vi "0008_FireEveryLastDayOfMonth.vi"(8 "error in (no error)":errorcluster) -> (0 "error out":errorcluster)   [LabVIEW 2013]
uses:
  <vilib>/addons/_JKI Toolkits/Caraya/classes/Assert/Assert True.vi
  source/Cron/Create Cron Expression.vi
  source/Cron/Compute Next Cron.vi
  source/Cron.Quartz/Cron.Quartz.lvclass
  <vilib>/addons/_JKI Toolkits/Caraya/classes/Test/Test.lvclass
  <vilib>/addons/_JKI Toolkits/Caraya/classes/Assert/Assert.lvclass
  source/openCron.lvlib
panel:
  out "Occurences":timestamp[](array[timestamp])
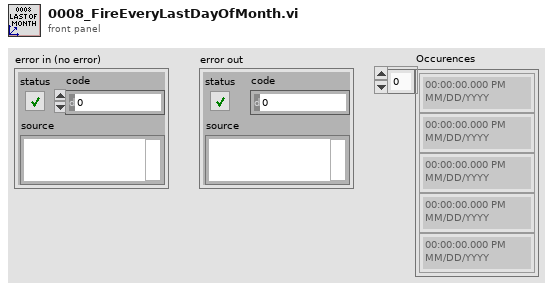
[diagram p1: front panel]
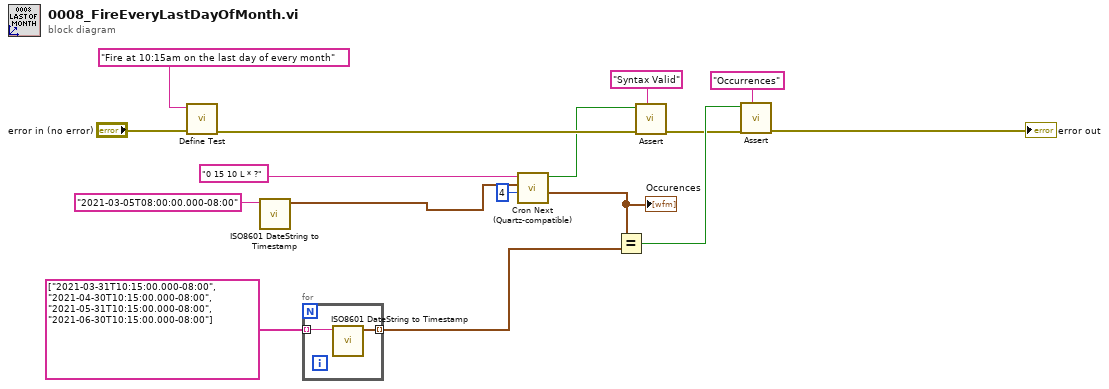
[diagram p0: block diagram]
diagram:
  n1 = call <vilib>:"Define Test.vi"("error in (no error)"="error in (no error)", "Label (VI Title)"="Fire at 10:15am on the last day of every month") -> ("error out"=w14:errorcluster)  [unwired: 8 in, 1 out]
  n2 = call <vilib>:"ISO8601 DateString to Timestamp.vi"("ISO8601 Date String"="2021-03-05T08:00:00.000-08:00" ("Expression")) -> ("Timestamp"=w2:timestamp)  [unwired: 8 in, 2 out]
  n3 = for {
    tunnel: string[] ["2021-03-31T10:15:00.000-08:00", "2021-04-30T10:15:00.000-08:00", "2021-05-31T10:15:00.000-08:00", "2021-06-30T10:15:00.000-08:00"] -> [w18] mode=indexing
    tunnel: [w17] -> w1 mode=indexing
    n4 = call <vilib>:"ISO8601 DateString to Timestamp.vi"("ISO8601 Date String"=w18) -> ("Timestamp"=w17:timestamp)  [unwired: 8 in, 2 out]
  }
  n5 = call "Cron Next (Quartz-compatible).vi"("Nb Occurences (min: 1)"=u16 4, "Reference timestamp (Now)"=w2, "Cron Expression"="0 15 10 L * ?" ("Expression")) -> ("Occurences"=w10:timestamp[], "syntax valid?"=w11:bool)  [unwired: 6 in, 1 out]
  "Occurences" <- w10
  n6 = Equal?(x=w10, y=w1) -> (x = y?=w13:bool)
  n7 = call-poly <vilib>:"Assert.vi"("Label"="Syntax Valid" ("Label (VI Title)"), "error in (no error)"=w14, "True?"=w11) -> ("error out"=w12:errorcluster)  [unwired: 7 in, 1 out]
  n8 = call-poly <vilib>:"Assert.vi"("Label"="Occurrences" ("Label (VI Title)"), "error in (no error)"=w12, "True?"=w13) -> ("error out"=→"error out":errorcluster)  [unwired: 7 in, 1 out]
